vi "Port To Atten Map.vi"(6 "Port":i32, 8 "error in":errorcluster) -> (0 "error out":errorcluster, 4 "txatten-sel":i32)   [LabVIEW 2018]
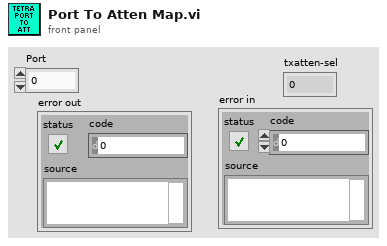
[diagram p1: front panel]
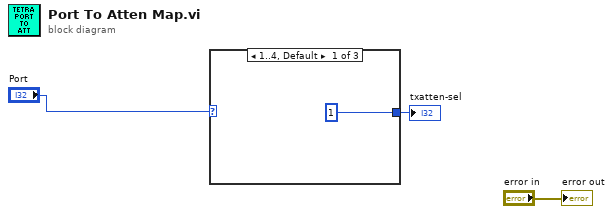
[diagram p0: block diagram]
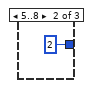
[diagram p2: hidden frame]
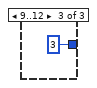
[diagram p3: hidden frame]
diagram:
  n1 = case shown="1..4, Default" "Port" {
    tunnel: [1 2 3] -> w3
    frame 1..4, Default {
    }
    frame 5..8 {
    }
    frame 9..12 {
    }
  }
  "txatten-sel" <- w3
  "error out" <- "error in"
